vi "Read_LL_Pressure.vi"() -> (3 "LL Pressure":dbl)   [LabVIEW 2014]
uses:
  <vilib>/Instr/_visa.llb/VISA Configure Serial Port (Instr).vi
panel:
  out "read buffer":string
  in  "baud rate (9600)":u32=19200
  in  "termination char\n(0xA = '\\n' = LF)":u8=13 format="%.0x"
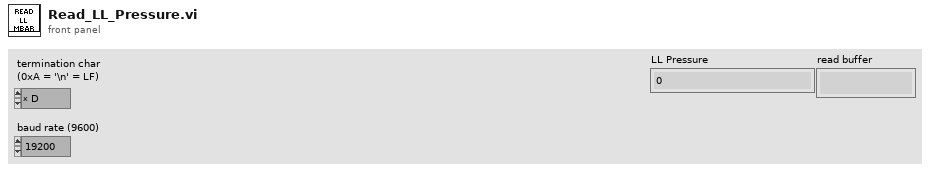
[diagram p1: front panel]
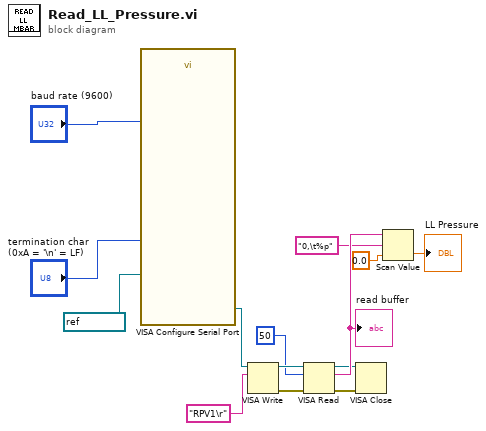
[diagram p0: block diagram]
diagram:
  n1 = call-poly "VISA Configure Serial Port"("VISA resource name"=refnum<visa-resource-name> "COM7", "termination char\n(0xA = '\\n' = LF)"="termination char\n(0xA = '\\n' = LF)", "baud rate (9600)"="baud rate (9600)") -> ("VISA resource name out"=w11:refnum<visa-resource-name>)  [unwired: 11 in, 1 out]
  n2 = VISA Write(VISA resource name=w11, write buffer="RPV1\r") -> (VISA resource name out=w9:refnum<visa-resource-name>, error out=w8:errorcluster)  [unwired: 1 in, 1 out]
  n3 = VISA Read(VISA resource name=w9, byte count=u32 50, error in (no error)=w8) -> (VISA resource name out=w2:refnum<visa-resource-name>, read buffer=w6:string, error out=w1:errorcluster)  [unwired: 1 out]
  "read buffer" <- w6
  n4 = VISA Close(VISA resource name=w2, error in (no error)=w1) -> ()  [unwired: 1 out]
  n5 = Scan Value(string=w6, format string="0,\t%p", default (0 dbl)=0.0) -> (value=→"LL Pressure":dbl)  [unwired: 1 out]
